vi "LabVIEW结合知识库调用本地大模型.vi"() -> ()   [LabVIEW 2023, in "LabVIEW RAG.lvlib"]
uses:
  RAG_LV_API/LabVIEW RAG.lvlib
  labview-local-model/openai_message.ctl
  labview-local-model/chat-role.ctl
  labview-local-model/chat-completion req.ctl
  <vilib>/Utility/error.llb/Trim Whitespace One-Sided.vi
  labview-local-model/LabVIEW LLM.lvlib
  labview-ai-share/LabVIEW AI Base.lvlib
panel:
  in  "Manage VectorDB":bool
  in  "知识库名":string="NI-cDAQ"
  in  "Top K":u32=10
  in  "API Key":string
  in  "system prompt":string="请注意，当用户询问有关NI硬件（如cDAQ）的问题时，cDAQ-9219 与 NI-9219、\"NI 9219\" 或 \"NI-9219\" 指的是同一种硬件。" caption="System提示词"
  in  "Stream?":bool
  in  "temperature (default: 0.8)":dbl=0.8 format="%.1f"
  in  "max tokens (default: 4096)":u32=4096
  in  "Clear":bool
  in  "model URL":string="http://localhost:1234/v1"
  in  "Send":bool
  in  "Input":string="NI 9230有多少个模拟输入通道？"
  in  "选择本地模型":string(combo)="deepseek-r1-distill-qwen-7b"
  out "error out":errorcluster
  in  "STOP":bool
  out "对话":string
  # "LabVIEW调用本地大模型"
  # "参数"
  # "知识库相关参数"
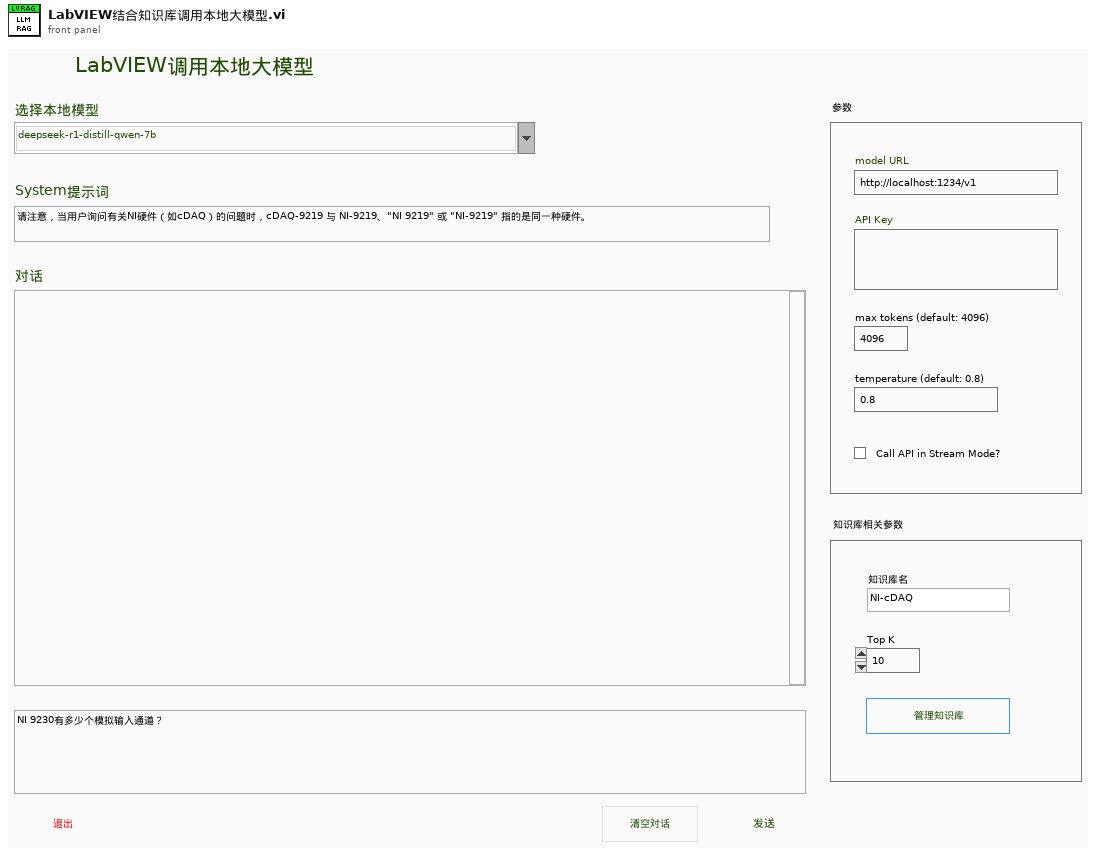
[diagram p1: front panel]
types:
  T1 = typedef "LabVIEW LLM.lvlib/openai_message.ctl" = cluster{"role":T2, "content":string, "reasoning":string}
  T2 = typedef "LabVIEW LLM.lvlib/chat-role.ctl" = enum16{"system", "user", "assistant"}
  T3 = typedef "LabVIEWHTTPClient.lvlib/ClientHandle.ctl" = refnum<k1>
  T4 = typedef "LabVIEW LLM.lvlib/chat-completion req.ctl" = cluster{"model":string, "messages":T1[], "max_tokens":u32, "temperature":dbl, "stream":bool, "reasoning":cluster{"effort":enum16{"high", "medium", "low"}, "exclude":bool}}
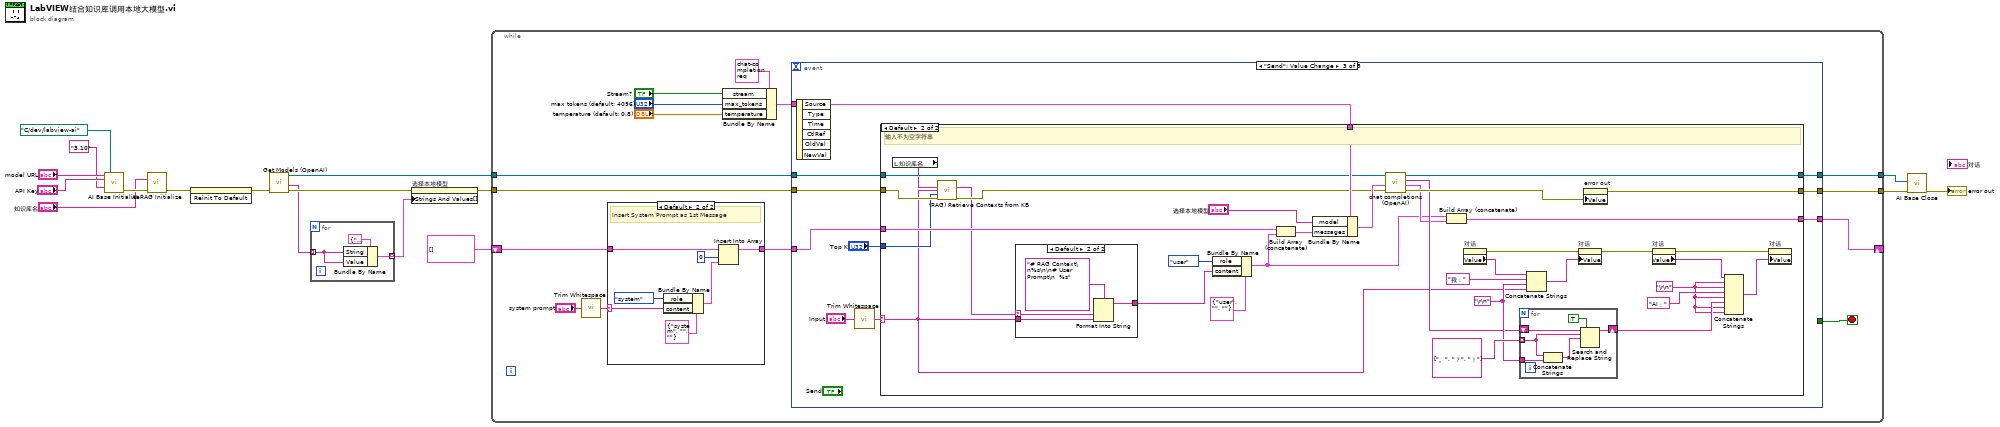
[diagram p0: block diagram]
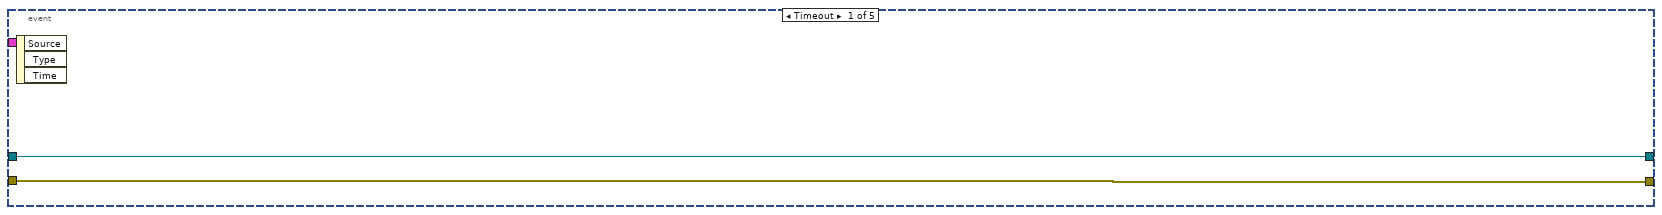
[diagram p3: hidden frame]
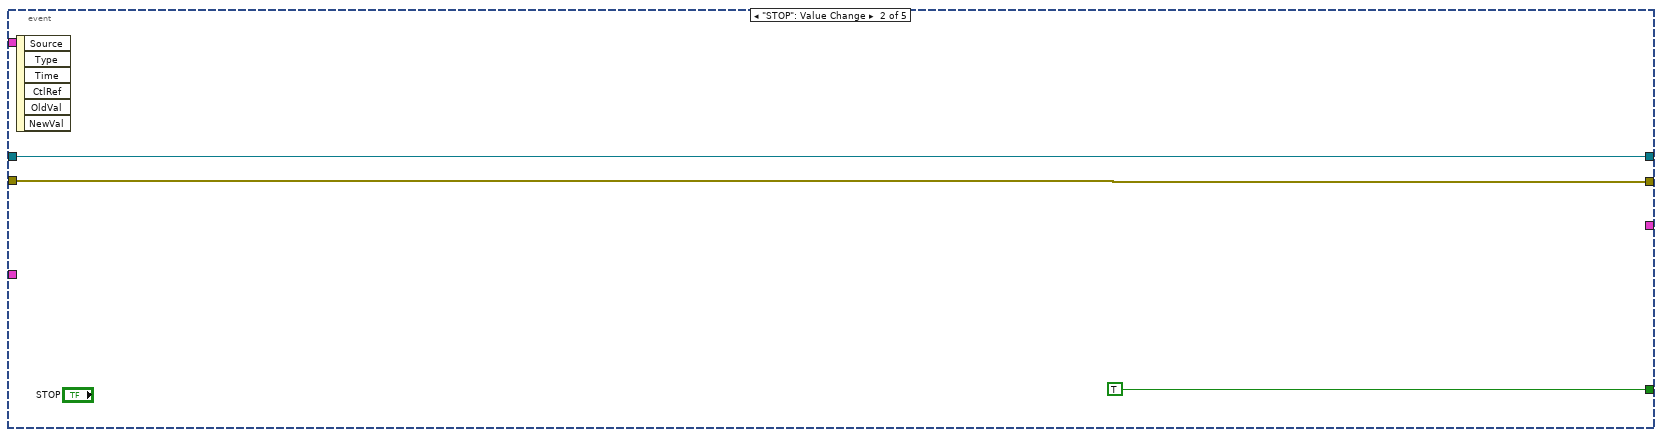
[diagram p4: hidden frame]
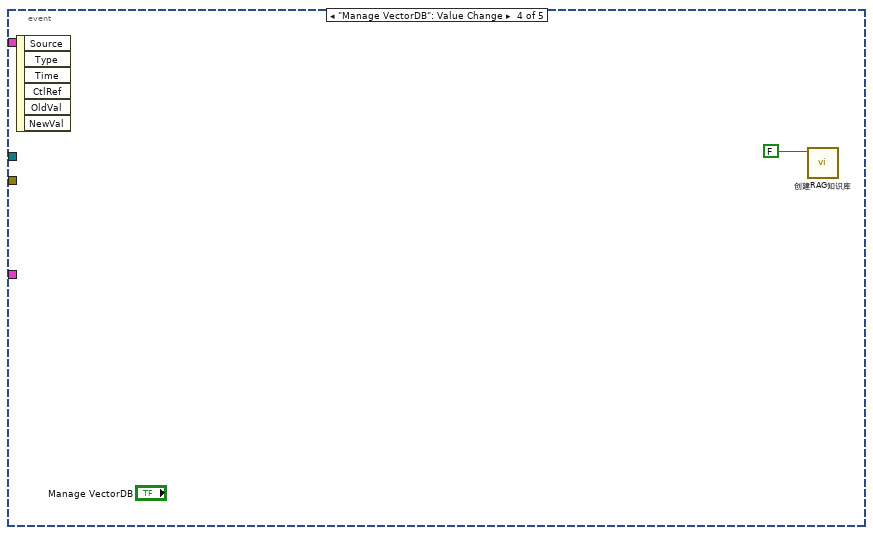
[diagram p7: hidden frame]
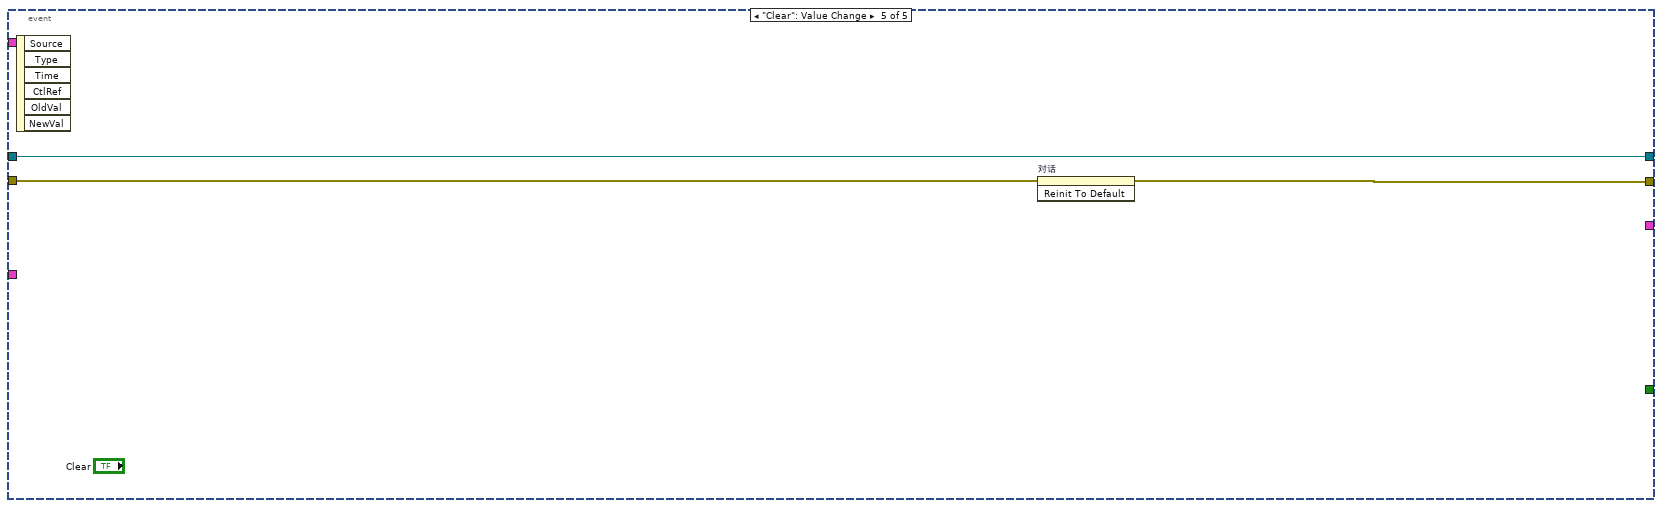
[diagram p8: hidden frame]
diagram:
  n1 = call "AI Base Initialize.vi"("OpenAI API URL"="model URL", "Python venv path"=path "C:/dev/labview-ai", "API Key"="API Key", "Python version"="3.10") -> ("error out"=w7:errorcluster)  [unwired: 9 in, 2 out]
  n2 = call "AI RAG Initialize.vi"("Knowledge Base Name"="知识库名", "error in (no error)"=w7) -> ("error out"=w4:errorcluster)  [unwired: 13 in]
  n3 = invoke on="Input" class="Str" method="Reinit To Default"(error in=w4) -> (error out=w9:errorcluster)  [unwired: 2 in, 2 out]
  n4 = call "Get Models (OpenAI).vi"("error in (no error)"=w9) -> ("error out"=w12:errorcluster, "Available Models"=w10:string[], "Refnum out"=w14:T3)  [unwired: 7 in, 1 out]
  n5 = for {
    tunnel: [w19] -> w13 mode=indexing
    tunnel: w10 -> [w18] mode=indexing
    n6 = Bundle By Name(cluster=cluster{"String":string, "Value":string} {"String"="", "Value"=""} ("Cluster"), "String"=w18, "Value"=w18) -> (w19:cluster{"String":string, "Value":string})
  }
  n7 = property on="选择本地模型" class="CmbBox"(error in=w12, "Strings And Values[]"=w13) -> (error out=w11:errorcluster)  [unwired: 1 in, 1 out]
  n8 = while {
    tunnel: w14 -> [w34]
    tunnel: w11 -> [w33]
    tunnel: [w32] -> w17
    tunnel: [w31] -> w16
    shift-right: [w30] -> _
    shift-left: T1[] [] ("previous messages") -> [w24]
    stop <- w35 stop-if-true
    n9 = call <vilib>:"Trim Whitespace.vi"("string"="system prompt") -> ("trimmed string"=w21:string)  [unwired: 1 in]
    n10 = case shown="Default" w21 {
      selector: w21 -> [_ w43]
      tunnel: w24 -> [w36 w38]
      tunnel: [w36 w40] -> w23
      frame "" {
      }
      frame Default {
        # "Insert System Prompt as 1st Message"
        n11 = Bundle By Name(cluster=T1 {"role"=enum."system", "content"="", "reasoning"=""} ("message"), "role"=enum16{"system", "user", "assistant"}."system", "content"=w43) -> (w39:T1)
        n12 = Insert Into Array(array=w38, index=0, new element=w39) -> (w40:T1[])
      }
    }
    n13 = Bundle By Name(cluster=T4 {"model"="", "messages"=[{"role"=enum."user", "content"="", "reasoning"=""}], "max_tokens"=4096, "temperature"=0.7, "stream"=FALSE, "reasoning"={"effort"=enum."low", "exclude"=FALSE}}, "stream"="Stream?", "max_tokens"="max tokens (default: 4096)", "temperature"="temperature (default: 0.8)") -> (w29:T4)
    n14 = event shown="[2] \"Send\": Value Change" {
      selector: _ -> [_ _ _ _ _]
      dyn-events: _ -> [_ _ _ _ _]
      timeout: _ -> [_ _ _ _ _]
      tunnel: [_ TRUE _ _ _] -> w35
      tunnel: w34 -> [w45 w47 w55 _ w111]
      tunnel: w33 -> [w44 w46 w57 _ w110]
      tunnel: w29 -> [_ _ w58 _ _]
      tunnel: [w45 w47 w56 _ w111] -> w32
      tunnel: [w44 w46 w54 _ w109] -> w31
      tunnel: [_ _ w52 _ _] -> w30
      tunnel: w23 -> [_ _ w51 _ _]
      event Timeout {
        n15 = event-data() -> ()  [unwired: 1 in, 3 out]
      }
      event "STOP": Value Change {
        n16 = event-data() -> ()  [unwired: 1 in, 6 out]
      }
      event "Send": Value Change {
        n17 = event-data() -> ()  [unwired: 1 in, 6 out]
        n18 = call <vilib>:"Trim Whitespace.vi"("string"="Input") -> ("trimmed string"=w50:string)  [unwired: 1 in]
        n19 = case shown="Default" w50 {
          selector: w50 -> [_ w63]
          tunnel: w58 -> [_ w96]
          tunnel: w57 -> [w61 w68]
          tunnel: [w60 w92] -> w56
          tunnel: w55 -> [w60 w91]
          tunnel: [w61 w90] -> w54
          tunnel: [w59 w73] -> w52
          tunnel: w51 -> [w59 w71]
          tunnel: "Top K" -> [_ w64]
          frame "" {
          }
          frame Default {
            w69 = "\r\n"
            w76 = "\r\n"
            # "输入不为空字符串"
            n20 = local read "知识库名"() -> (w62:string)
            n21 = call "(RAG) Retrieve Contexts from KB.vi"("Knowledge Base Name"=w62, "RAG Query"=w63, "K"=w64, "error in"=w68) -> ("Retrieved Contexts"=w66:string, "error out"=w67:errorcluster)  [unwired: 9 in, 1 out]
            n22 = case shown="Default" w66 {
              selector: w66 -> [_ w100]
              tunnel: [w97 w99] -> w65
              tunnel: w63 -> [w97 w98]
              frame "" {
              }
              frame Default {
                n23 = Format Into String(format string="# RAG Context\n%s\n\n# User Prompt\n  %s", w100, w98) -> (resulting string=w99:string)  [unwired: 2 in, 1 out]
              }
            }
            n24 = Bundle By Name(cluster=T1 {"role"=enum."user", "content"="", "reasoning"=""} ("messages"), "role"=enum16{"system", "user", "assistant"}."user", "content"=w65) -> (w72:T1)
            n25 = Build Array (concatenate)(w71, w72) -> (w93:T1[])
            n26 = Bundle By Name(cluster=w96, "model"="选择本地模型", "messages"=w93) -> (w95:T4)
            n27 = call "chat completions (OpenAI).vi"("error in"=w67, "chat-completion req"=w95, "Refnum in"=w91) -> ("error out"=w89:errorcluster, "previous messages"=w74:T1[], "Answer content"=w75:string, "Refnum out"=w92:T3)  [unwired: 4 in, 1 out]
            n28 = Build Array (concatenate)(w72, w74) -> (w73:T1[])
            n29 = property on="对话" class="Str"() -> (error out=w88:errorcluster, "Value"=w87:string)  [unwired: 2 in, 1 out]
            n30 = for {
              tunnel: string[] ["。", "？", "！"] ("search string") -> [w105] mode=indexing
              tunnel: w76 -> [w103]
              shift-right: [w107] -> w78
              shift-left: w75 -> [w102]
              n31 = Concatenate Strings(w105, w103) -> (w104:string)
              n32 = Search and Replace String(replace all?=TRUE ("replace all? (F)"), input string=w102, search string=w105, replace string=w104) -> (result string=w107:string)  [unwired: 4 in, 3 out]
            }
            n33 = Concatenate Strings(w87, "我：" ("string"), w76, w63) -> (w86:string)
            n34 = property on="对话" class="Str"(error in=w88, "Value"=w86) -> (error out=w81:errorcluster)  [unwired: 1 in, 1 out]
            n35 = property on="error out" class="Clust (strict)"("Value"=w89) -> (error out=w90:errorcluster)  [unwired: 2 in, 1 out]
            n36 = property on="对话" class="Str"(error in=w81) -> (error out=w82:errorcluster, "Value"=w79:string)  [unwired: 1 in, 1 out]
            n37 = Concatenate Strings(w79, w69, w69, "AI：" ("string"), w69, w78, w69, w69) -> (w80:string)
            n38 = property on="对话" class="Str"(error in=w82, "Value"=w80) -> ()  [unwired: 1 in, 2 out]
          }
        }
      }
      event "Manage VectorDB": Value Change {
        n39 = event-data() -> ()  [unwired: 1 in, 6 out]
        n40 = call "创建RAG知识库.vi"("init base£"=FALSE) -> ()  [unwired: 11 in]
      }
      event "Clear": Value Change {
        n41 = event-data() -> ()  [unwired: 1 in, 6 out]
        n42 = invoke on="对话" class="Str" method="Reinit To Default"(error in=w110) -> (error out=w109:errorcluster)  [unwired: 2 in, 2 out]
      }
    }
  }
  n43 = call "AI Base Close.vi"("error in"=w16, "Http Refnum in"=w17) -> ("error out"=→"error out":errorcluster)  [unwired: 9 in]
